vi "Check.vi"(8 "error in (no error)":errorcluster, 11 "Notifier in":refnum<class "Notifier.lvclass">) -> (0 "error out":errorcluster, 3 "Notifier is valid?":bool)   [LabVIEW 2020, in "Data.lvlib" / "Notifier.lvclass"]
doc: "Check if the notifier is valid."
uses:
  Notifier.lvclass
  Notifier.lvclass/Notifier.ctl
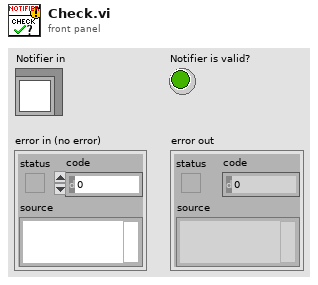
[diagram p1: front panel]
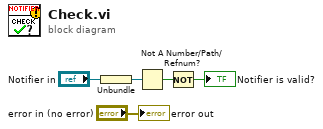
[diagram p0: block diagram]
diagram:
  n1 = Unbundle("Notifier in") -> (w3:refnum<notifier>)
  n2 = Not A Number/Path/Refnum?(number/path/refnum=w3) -> (NaN/Path/Refnum?=w2:bool)
  n3 = Not(x=w2) -> (.not. x?=→"Notifier is valid?":bool)
  "error out" <- "error in (no error)"
